vi "TestManyPublications.vi"(8 "error in (no error)":errorcluster, 11 "TestPublishRate In":refnum<class "TestManyPublications.lvclass">) -> (0 "error out":errorcluster, 3 "TestPublishRate Out":refnum<class "TestManyPublications.lvclass">)   [LabVIEW 2020, in "TestFrameworkPerformance.lvlib" / "TestManyPublications.lvclass"]
uses:
  TestManyPublications.lvclass
  TestManyPublications.lvclass/TestManyPublications.ctl
  Source/IViewModel/IViewModel/IViewModel.lvclass
  Source/IViewable/IViewable/IViewable.lvclass
  <vilib>/ActorFramework/Actor/Actor.lvclass
  modules/mva-core/Source/SubscriptionPolicy/ValueChangeSubscription/ValueChangeSubscription.lvclass
  modules/mva-core/Source/IMediator/SubscriptionRequest/SubscriptionRequest.lvclass
  modules/mva-core/Source/IMediator/ISubscriptionPolicy/ISubscriptionPolicy.lvclass
  modules/mva-core/Source/Mediator/Mediator/Mediator.lvclass
  modules/mva-core/Source/IObserver/IObserver Messages/Subscribe Msg/Subscribe Msg.lvclass
  <vilib>/ActorFramework/Stop Msg/Stop Msg.lvclass
  TestModelManyTopics/TestModelManyTopics.lvclass
  81cf93a4-50d8-414a-8355-1077334c3962.vi
  540f04fc-0b85-431b-8f57-02b9bbd5a47e.vi
  modules/composed-transport/Source/Concrete/QueueTransport/QueueTransport.lvclass
  C:/Git/mva-viewable/modules/mva-core/Source/IMediator/ISubscriptionPolicy/ISubscriptionPolicy.lvclass
  C:/Git/mva-viewable/modules/mva-core/Source/SubscriptionPolicy/ValueChangeSubscription/ValueChangeSubscription.lvclass
  C:/Git/mva-viewable/modules/composed-transport/Source/ITransport/ITransport.lvclass
  C:/Git/mva-viewable/modules/composed-transport/Source/Concrete/QueueTransport/QueueTransport.lvclass
  C:/Git/mva-viewable/Source/IViewManager/IViewManager/IViewManager.lvclass
  C:/Git/mva-viewable/Source/IViewable/IViewable/IViewable.lvclass
  C:/Git/mva-viewable/Source/ActorEvents/IEventAggregator/IEventAggregator.lvclass
  C:/Git/mva-viewable/modules/mva-core/Source/IObserver/IObserver/IObserver.lvclass
  C:/Program Files (x86)/National Instruments/LabVIEW 2020/vi.lib/ActorFramework/Actor/Actor.lvclass
  C:/Git/mva-viewable/Source/IViewModel/IViewModel/IViewModel.lvclass
panel:
  out "Final Sample Transmission Time":dbl
  out "1Hz Cycle Transmission Times":dbl[](graph)
  out "Iteration":i32
  # "LV 2015 (no in-place VAT read) -- 0.53 sec typical\nLV 2017 (in-place VAT get element) -- 0.02 to 0.03 sec typical\nLV 2017 (In-place Transport) -- 0.0065 sec typical (with debug log = True)"
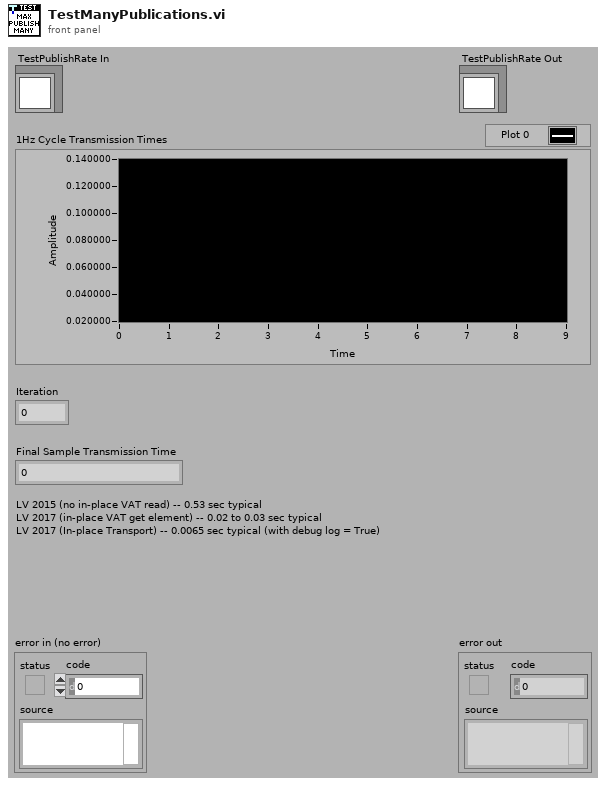
[diagram p1: front panel]
types:
  T1 = typedef "IMediator.lvlib/ISubscriptionPolicy.lvclass/ISubscriptionPolicy Reference.ctl" = refnum<data-value>
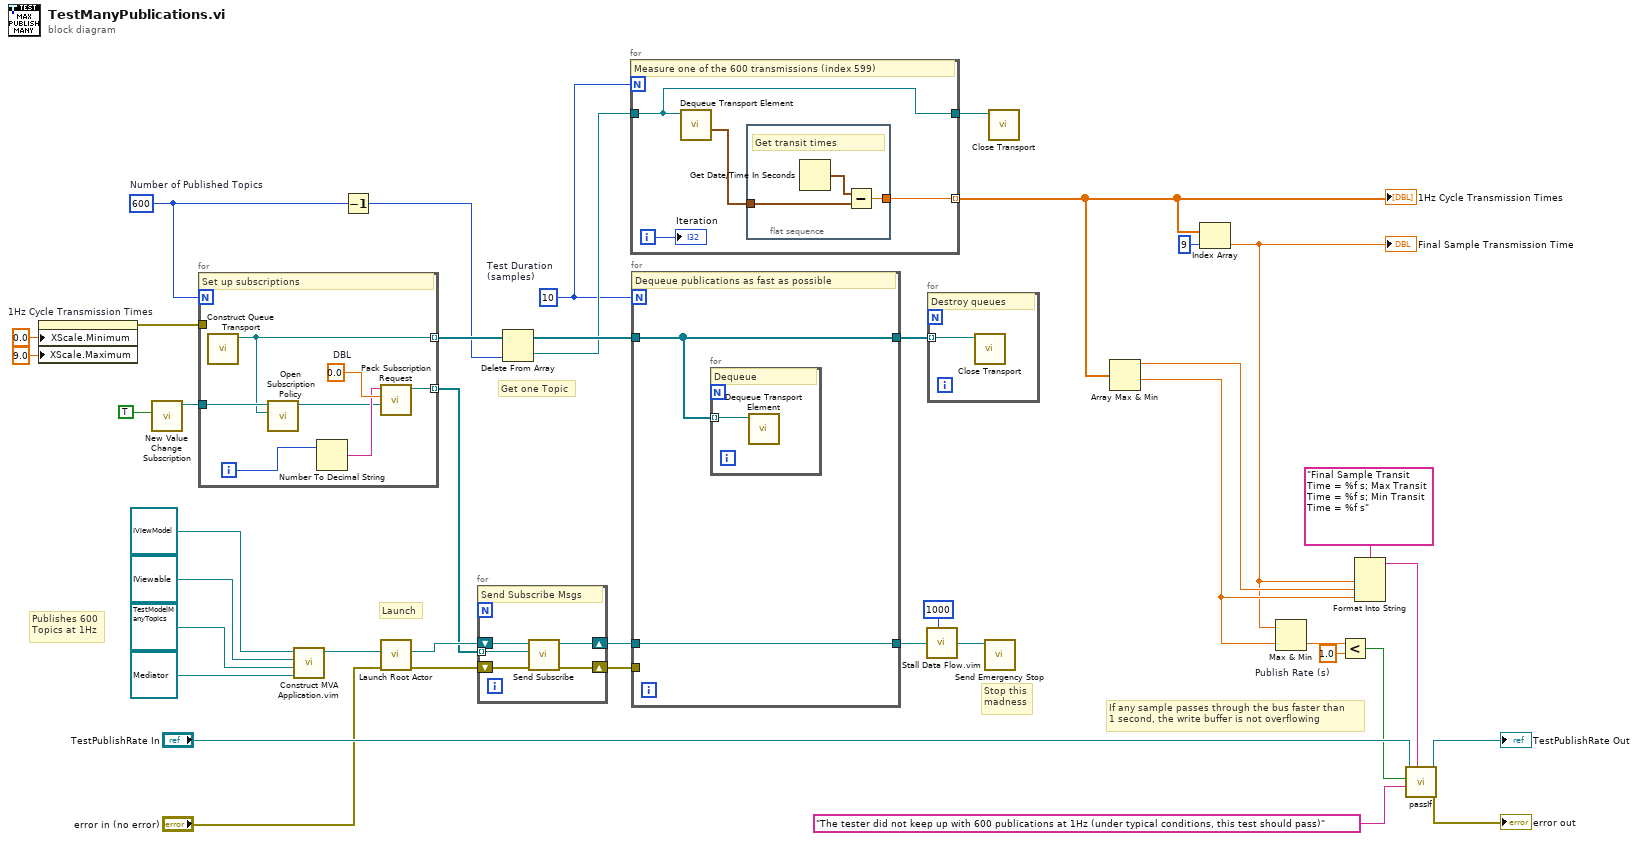
[diagram p0: block diagram]
diagram:
  w9 = 1.0  # Publish Rate (s)
  w7 = 600  # Number of Published Topics
  w17 = 10  # Test Duration (samples)
  # "Publishes 600\nTopics at 1Hz"
  # "If any sample passes through the bus faster than\n1 second, the write buffer is not overflowing"
  # "Get one Topic"
  # "Stop this\nmadness"
  # "Launch"
  n1 = property on="1Hz Cycle Transmission Times" class="WFChart (strict)"("XScale.Minimum"=0.0 ("X Scale.Range:Minimum"), "XScale.Maximum"=9.0 ("X Scale.Range:Maximum")) -> (error out=w1:errorcluster)  [unwired: 2 in, 1 out]
  n2 = call "New Value Change Subscription.vi"("Ignore Past Updates? (F)"=TRUE) -> ("ValueChangeSubscription Out"=w22:refnum<class "ValueChangeSubscription.lvclass">)  [unwired: 10 in]
  n3 = for {
    N: w7 -> [_]
    tunnel: [w48] -> w31 mode=indexing
    tunnel: w22 -> [w46]
    tunnel: [w43] -> w21 mode=indexing
    tunnel: w1 -> [_]
    i -> [w45]
    w47 = 0.0  # DBL
    # "Set up subscriptions"
    n4 = call "Construct Queue Transport.vi"() -> ("QueueTransport"=w43:refnum<class "QueueTransport.lvclass">)  [unwired: 10 in, 1 out]
    n5 = call "Open Subscription Policy.vi"("Transport"=w43, "SubscriptionPolicy"=w46) -> ("Subscription Policy"=w42:T1)  [unwired: 8 in, 1 out]
    n6 = Number To Decimal String(number=w45) -> (decimal integer string=w44:string)  [unwired: 1 in]
    n7 = call "Pack Subscription Request.vi"("Subscription Policy"=w42, "Type"=w47, "Datum Name"=w44) -> ("SubscriptionRequest"=w48:refnum<class "SubscriptionRequest.lvclass">)  [unwired: 7 in, 1 out]
  }
  n8 = call "Construct MVA Application.vim"("Mediator Type"=refnum<class "Mediator.lvclass"> refnum ("Mediator"), "Model Type"=refnum<class "TestModelManyTopics.lvclass"> refnum ("Model"), "Startup View Configuration"=refnum<class "IViewable.lvclass"> refnum, "IViewModel In"=refnum<class "IViewModel.lvclass"> refnum) -> ("IViewModel Out"=w33:refnum<class "IViewModel.lvclass">)  [unwired: 7 in]
  n9 = Decrement(x=w7) -> (x-1=w6:i32)
  n10 = call <vilib>:"Launch Root Actor.vi"("error in (no error)"="error in (no error)", "Actor"=w33) -> ("error out"=w29:errorcluster, "Actor's Enqueuer"=w32:refnum<class "Message Enqueuer.lvclass">)  [unwired: 8 in]
  n11 = for {
    tunnel: w31 -> [w52] mode=indexing
    shift-right: [w51] -> w30
    shift-left: w32 -> [w53]
    shift-right: [w49] -> w28
    shift-left: w29 -> [w50]
    # "Send Subscribe Msgs"
    n12 = call "Send Subscribe.vi"("error in (no error)"=w50, "SubscriptionRequest"=w52, "Message Enqueuer"=w53) -> ("error out"=w49:errorcluster, "Message Enqueuer out"=w51:refnum<class "Message Enqueuer.lvclass">)  [unwired: 7 in]
  }
  n13 = Delete From Array(array=w21, index=w6) -> (deleted portion=w19:refnum<class "QueueTransport.lvclass">, array with subset deleted=w20:refnum<class "QueueTransport.lvclass">[])  [unwired: 1 in]
  n14 = for {
    N: w17 -> [_]
    tunnel: w19 -> [w54]
    tunnel: [w54] -> w18
    tunnel: [w57] -> w14 mode=indexing
    i -> [w56]
    # "Measure one of the 600 transmissions (index 599)"
    n15 = call "Dequeue Transport Element.vi"("QueueTransport"=w54) -> ("Publication Time"=w55:timestamp)  [unwired: 7 in, 3 out]
    n16 = flat-sequence {
      tunnel: [w59] -> w57
      tunnel: w55 -> [w58]
      frame #0 {
        # "Get transit times"
        n17 = Get Date/Time In Seconds() -> (seconds since 1Jan1904=w60:timestamp)
        n18 = Subtract(x=w60, y=w58) -> (x-y=w59:dbl)
      }
    }
    "Iteration" <- w56
  }
  "1Hz Cycle Transmission Times" <- w14
  n19 = for {
    N: w17 -> [_]
    tunnel: w30 -> [w62]
    tunnel: w28 -> [_]
    tunnel: [w62] -> w27
    tunnel: [w61] -> w26
    tunnel: w20 -> [w61]
    # "Dequeue publications as fast as possible"
    n20 = for {
      tunnel: w61 -> [w63] mode=indexing
      # "Dequeue"
      n21 = call "Dequeue Transport Element.vi"("QueueTransport"=w63) -> ()  [unwired: 7 in, 4 out]
    }
  }
  n22 = call "Stall Data Flow.vim"("value in"=w27, "milliseconds to wait"=u32 1000) -> ("value out"=w5:refnum<class "Message Enqueuer.lvclass">)  [unwired: 1 out]
  n23 = for {
    tunnel: w26 -> [w64] mode=indexing
    # "Destroy queues"
    n24 = call-dynamic "Close Transport.vi"("QueueTransport"=w64) -> ()  [unwired: 10 in, 1 out]
  }
  n25 = call <vilib>:"Send Emergency Stop.vi"("Message Enqueuer"=w5) -> ()  [unwired: 10 in, 1 out]
  n26 = call-dynamic "Close Transport.vi"("QueueTransport"=w18) -> ()  [unwired: 10 in, 1 out]
  n27 = Array Max & Min(array=w14) -> (max value=w13:dbl, min value=w12:dbl)  [unwired: 2 out]
  n28 = Index Array(array=w14, index=9) -> (element=w11:dbl)
  "Final Sample Transmission Time" <- w11
  n29 = Max & Min(x=w11, y=w12) -> (min(x,y)=w10:dbl)  [unwired: 1 out]
  n30 = Less?(x=w10, y=w9) -> (x < y?=w8:bool)
  n31 = Format Into String(format string="Final Sample Transit Time = %f s; Max Transit Time = %f s; Min Transit Time = %f s", w11, w13, w12) -> (resulting string=w25:string)  [unwired: 2 in, 1 out]
  n32 = call-dynamic "passIf.vi"("custom report message (\"\")"=w25, "message (\"\")"="The tester did not keep up with 600 publications at 1Hz (under typical conditions, this test should pass)" ("message (\"\")"), "pass"=w8, "TestCase in"="TestPublishRate In") -> ("error out"=→"error out":errorcluster, "TestCase out"=→"TestPublishRate Out":refnum<class "TestManyPublications.lvclass">)  [unwired: 6 in]
